vi "Single Read.vi"() -> ()   [LabVIEW 2023]
uses:
  <vilib>/Analysis/2dsp.llb/Complex FFT.vi
  VIs/Initialize by Serial.vi
  RTL-SDR.lvlib
  <vilib>/Analysis/NI_AALPro.lvlib
panel:
  out "error out":errorcluster
  in  "FFT size":i32=8192
  out "# Samples":i32
  out "FFT Graph":cluster{"f0":dbl, "df":dbl, "Y":dbl[]}(graph)
  out "Actual Sample Rate (Hz)":u32 format="%#.6p"
  in  "Sample Rate (Hz)":u32=2000000 format="%#.6p"
  out "Manufacturer Name":string
  out "Product Name":string
  out "Serial Number":string
  in  "Center Frequency (Hz)":u32=80000000 format="%#_6p"
  out "Actual Center Frequency (Hz)":u32 format="%#.6p"
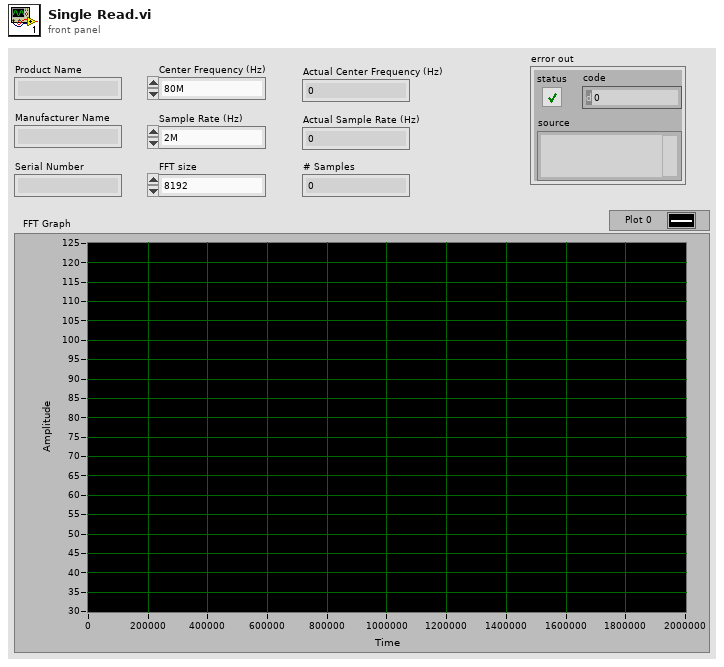
[diagram p1: front panel]
types:
  T1 = typedef "RTL-SDR.lvlib/Device Handle.ctl" = u64
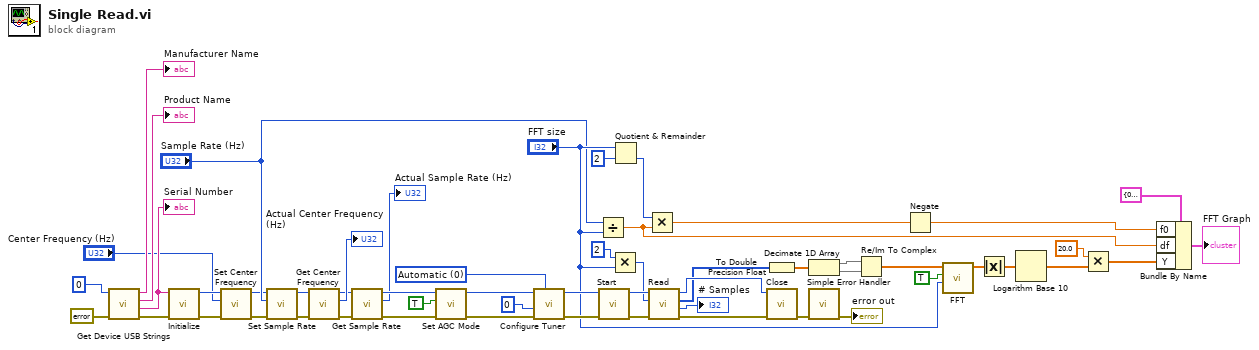
[diagram p0: block diagram]
diagram:
  w32 = u16 0 items=["Automatic", "Manual"] ("Tuner Gain Mode")
  n1 = call "Get Device USB Strings.vi"("error in (no error)"=errorcluster {"status"=FALSE, "code"=0, "source"=""} ("error in"), "device index"=u32 0) -> ("error out"=w54:errorcluster, "Serial Number"=w50:string, "Product Name"=→"Product Name":string, "Manufacturer Name"=→"Manufacturer Name":string)  [unwired: 6 in]
  "Serial Number" <- w50
  n2 = call-poly "Initialize.vi"("error in (no error)"=w54, "Serial Number"=w50) -> ("error out"=w46:errorcluster, "device handle out"=w47:T1)  [unwired: 8 in]
  n3 = call "Set Center Frequency.vi"("error in (no error)"=w46, "Center Frequency (Hz)"="Center Frequency (Hz)", "device handle in"=w47) -> ("error out"=w6:errorcluster, "device handle out"=w7:T1)  [unwired: 7 in]
  n4 = call "Set Sample Rate.vi"("error in (no error)"=w6, "Sample Rate (Hz)"="Sample Rate (Hz)", "device handle in"=w7) -> ("error out"=w39:errorcluster, "device handle out"=w38:T1)  [unwired: 7 in]
  n5 = call "Get Center Frequency.vi"("error in (no error)"=w39, "device handle in"=w38) -> ("error out"=w8:errorcluster, "Center Frequency (Hz)"=→"Actual Center Frequency (Hz)":u32, "device handle out"=w9:T1)  [unwired: 7 in]
  n6 = call "Get Sample Rate.vi"("error in (no error)"=w8, "device handle in"=w9) -> ("error out"=w29:errorcluster, "Sample Rate (Hz)"=→"Actual Sample Rate (Hz)":u32, "device handle out"=w30:T1)  [unwired: 7 in]
  n7 = call "Set AGC Mode.vi"("error in (no error)"=w29, "Enable AGC (T)"=TRUE, "device handle in"=w30) -> ("error out"=w35:errorcluster, "device handle out"=w34:T1)  [unwired: 7 in]
  n8 = call "Configure Tuner.vi"("Tuner Gain Mode (0: auto)"=w32, "error in (no error)"=w35, "Bandwidth (Hz) (0: auto)"=u32 0, "device handle in"=w34) -> ("error out"=w27:errorcluster, "device handle out"=w28:T1)  [unwired: 6 in]
  n9 = Divide(x="Sample Rate (Hz)", y="FFT size") -> (x/y=w3:dbl)
  n10 = call "Start.vi"("error in (no error)"=w27, "device handle in"=w28) -> ("error out"=w42:errorcluster, "device handle out"=w43:T1)  [unwired: 8 in]
  n11 = Multiply(x=2, y="FFT size") -> (x*y=w41:i32)
  n12 = Quotient & Remainder(x="FFT size", y=2) -> (floor(x/y)=w12:i32)  [unwired: 1 out]
  n13 = Multiply(x=w12, y=w3) -> (x*y=w13:dbl)
  n14 = call "Read.vi"("error in (no error)"=w42, "# Samples to read"=w41, "device handle in"=w43) -> ("error out"=w48:errorcluster, "Actual # Samples"=→"# Samples":i32, "Samples"=w10:u8[], "device handle out"=w49:T1)  [unwired: 5 in]
  n15 = To Double Precision Float(number=w10) -> (double precision float=w21:dbl[])
  n16 = call "Close.vi"("error in"=w48, "device handle in"=w49) -> ("error out"=w45:errorcluster)  [unwired: 9 in]
  n17 = Decimate 1D Array(w21) -> (w20:dbl[], w19:dbl[])
  n18 = call <vilib>:"Simple Error Handler.vi"("error in (no error)"=w45) -> ("error out"=→"error out":errorcluster)  [unwired: 4 in, 4 out]
  n19 = Re/Im To Complex(1:w19, 2:w20) -> (0:w18:cdb[])
  n20 = Negate(x=w13) -> (-x=w4:dbl)
  n21 = call-poly <vilib>:"FFT.vi"("FFT size"="FFT size", "shift?"=TRUE, "X"=w18) -> ("FFT {X}"=w23:cdb[])  [unwired: 7 in, 1 out]
  n22 = Absolute Value(x=w23) -> (abs(x)=w15:dbl[])
  n23 = Logarithm Base 10(1:w15) -> (0:w17:dbl[])
  n24 = Multiply(x=20.0, y=w17) -> (x*y=w2:dbl[])
  n25 = Bundle By Name(cluster=cluster{"f0":dbl, "df":dbl, "Y":dbl[]} {"f0"=0.0, "df"=0.0, "Y"=[]}, "f0"=w4, "df"=w3, "Y"=w2) -> (→"FFT Graph":cluster{"f0":dbl, "df":dbl, "Y":dbl[]})
